vi "DeadbandJoystick.vi"(9 "Z":dbl, 10 "Y":dbl, 11 "X":dbl) -> (3 "SpeedOutput":dbl[](array[numeric]))   [LabVIEW 2018]
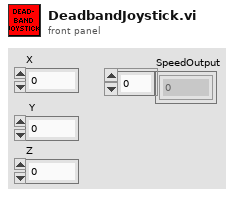
[diagram p1: front panel]
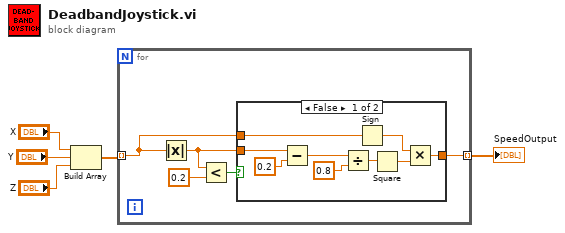
[diagram p0: block diagram]
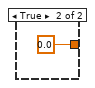
[diagram p2: hidden frame]
diagram:
  n1 = Build Array("X", "Y", "Z") -> (w4:dbl[])
  n2 = for {
    tunnel: w4 -> [w7] mode=indexing
    tunnel: [w6] -> w5 mode=indexing
    n3 = Absolute Value(x=w7) -> (abs(x)=w8:dbl)
    n4 = Less?(x=w8, y=0.2) -> (x < y?=w10:bool)
    n5 = case shown="False" w10 {
      tunnel: w8 -> [w19 _]
      tunnel: [w11 0.0] -> w6
      tunnel: w7 -> [w14 _]
      frame False {
        n6 = Subtract(x=w19, y=0.2) -> (x-y=w17:dbl)
        n7 = Divide(x=w17, y=0.8) -> (x/y=w15:dbl)
        n8 = Sign(1:w14) -> (0:w12:dbl)
        n9 = Square(x=w15) -> (x^2=w13:dbl)
        n10 = Multiply(x=w12, y=w13) -> (x*y=w11:dbl)
      }
      frame True {
      }
    }
  }
  "SpeedOutput" <- w5
